vi "Distance.vi"(1 "y2":dbl, 2 "x2":dbl, 3 "y1":dbl, 4 "x1":dbl) -> (0 "dist":dbl)   [LabVIEW 2017]
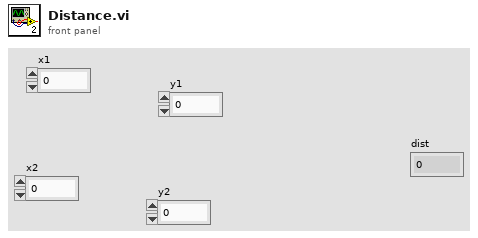
[diagram p1: front panel]
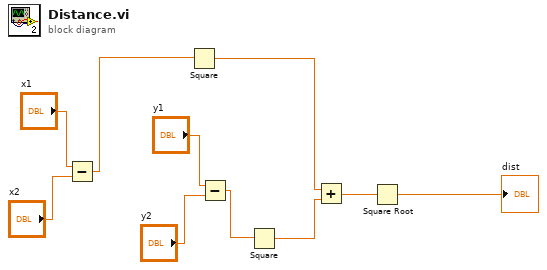
[diagram p0: block diagram]
diagram:
  n1 = Subtract(x="x1", y="x2") -> (x-y=w6:dbl)
  n2 = Square(x=w6) -> (x^2=w5:dbl)
  n3 = Subtract(x="y1", y="y2") -> (x-y=w4:dbl)
  n4 = Square(x=w4) -> (x^2=w3:dbl)
  n5 = Add(x=w5, y=w3) -> (x+y=w2:dbl)
  n6 = Square Root(x=w2) -> (sqrt(x)=→"dist":dbl)
